vi "Mask Write Holding Register.vi"(4 "OR mask":u16, 6 "AND mask":u16, 8 "error in (no error)":errorcluster, 10 "address":u16, 11 "Modbus master in":refnum<class "Modbus Master.lvclass">) -> (0 "error out":errorcluster, 3 "Modbus master out":refnum<class "Modbus Master.lvclass">)   [LabVIEW 2020, in "Modbus Master.lvclass"]
doc: "Writes values to one or more bits of a holding register."
uses:
  <vilib>/Modbus/master/Modbus Master.lvclass
  C:/builds/penguin/iak/lvdsc/trunk/20.0/lv/vi.lib/Modbus/subvis/Modbus API/Modbus API.lvclass
  <vilib>/Modbus/subvis/Modbus API/Modbus API.lvclass/Modbus API.ctl
  <vilib>/Modbus/master/Modbus Master.lvclass/Modbus Master.ctl
  <vilib>/Modbus/subvis/Protocol/Interfaces/Network Master/Network Master.lvclass
  C:/builds/penguin/iak/lvdsc/trunk/20.0/lv/vi.lib/Modbus/subvis/Protocol/Interfaces/Network Protocol/Network Protocol.lvclass
  <vilib>/Modbus/subvis/Transmission Data Unit (ADU)/Transmission Data Unit/Transmission Data Unit.lvclass
  <vilib>/Modbus/subvis/Data and Functions/Master Function Definition/Master Function Definition.lvlib
  <vilib>/Modbus/subvis/Modbus API/Modbus API.lvclass
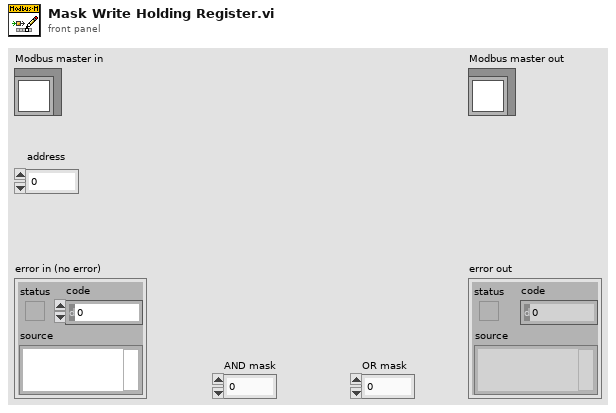
[diagram p1: front panel]
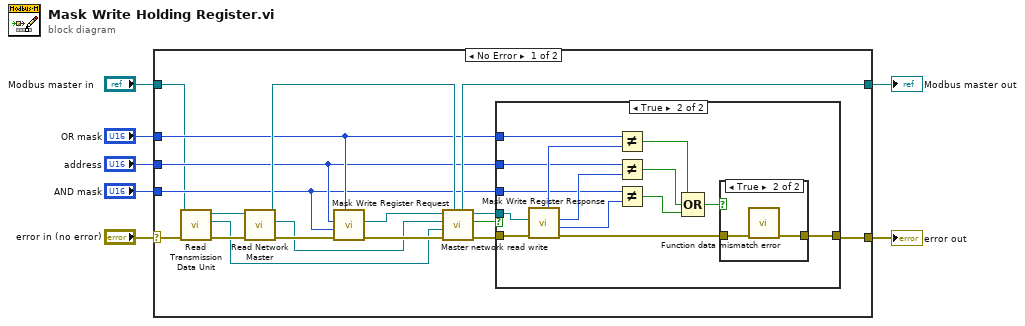
[diagram p0: block diagram]
diagram:
  n1 = case shown="No Error" "error in (no error)" {
    selector: "error in (no error)" -> [w8 w44]
    tunnel: "Modbus master in" -> [w9 w45]
    tunnel: [w19 w45] -> w6
    tunnel: [w23 w44] -> w5
    tunnel: "OR mask" -> [w13 _]
    tunnel: "address" -> [w12 _]
    tunnel: "AND mask" -> [w11 _]
    frame No Error {
      n2 = call <vilib>:"Read Transmission Data Unit.vi"("error in (no error)"=w8, "Modbus instance in"=w9) -> ("error out"=w17:errorcluster, "transmission data unit"=w15:refnum<class "Transmission Data Unit.lvclass">, "Modbus instance out"=w18:refnum<class "Modbus Master.lvclass">)  [unwired: 7 in]
      n3 = call <vilib>:"Read Network Master.vi"("error in (no error)"=w17, "Modbus master in"=w18) -> ("error out"=w16:errorcluster, "network master"=w14:refnum<class "Network Master.lvclass">, "Modbus master out"=w25:refnum<class "Modbus Master.lvclass">)  [unwired: 7 in]
      n4 = call <vilib>:"Mask Write Register Request.vi"("OR mask"=w13, "error in (no error)"=w16, "AND mask"=w11, "starting address"=w12) -> ("error out"=w24:errorcluster, "Modbus data unit out"=w21:refnum<class "Modbus Data Unit (PDU).lvclass">)  [unwired: 6 in]
      n5 = call <vilib>:"Master network read write.vi"("Modbus master in"=w25, "error in (no error)"=w24, "transmission data unit in"=w15, "network master in"=w14, "Modbus data unit in"=w21) -> ("error out"=w22:errorcluster, "PDU valid?"=w10:bool, "Modbus data unit out"=w20:refnum<class "Modbus Data Unit (PDU).lvclass">, "Modbus master out"=w19:refnum<class "Modbus Master.lvclass">)  [unwired: 3 in]
      n6 = case shown="True" w10 {
        tunnel: [w26 w38] -> w23
        tunnel: w22 -> [w26 w35]
        tunnel: w20 -> [_ w34]
        tunnel: w13 -> [_ w29]
        tunnel: w11 -> [_ w28]
        tunnel: w12 -> [_ w27]
        frame False {
        }
        frame True {
          n7 = call <vilib>:"Mask Write Register Response.vi"("error in (no error)"=w35, "Modbus data unit in"=w34) -> ("error out"=w33:errorcluster, "AND mask"=w36:u16, "address"=w37:u16, "OR mask"=w30:u16)  [unwired: 6 in]
          n8 = Not Equal?(x=w29, y=w30) -> (x != y?=w31:bool)
          n9 = Not Equal?(x=w27, y=w37) -> (x != y?=w32:bool)
          n10 = Not Equal?(x=w28, y=w36) -> (x != y?=w40:bool)
          n11 = Compound Arithmetic op=OR(w31, w32, w40) -> (w39:bool)
          n12 = case shown="True" w39 {
            tunnel: [w41 w43] -> w38
            tunnel: w33 -> [w41 w42]
            frame False {
            }
            frame True {
              n13 = call <vilib>:"Function data mismatch error.vi"("error in (no error)"=w42) -> ("error out"=w43:errorcluster)  [unwired: 10 in]
            }
          }
        }
      }
    }
    frame Error {
    }
  }
  "error out" <- w5
  "Modbus master out" <- w6
